vi "WPI_AccumulatorToVoltageSeconds.vi"(8 "error in (no error)":errorcluster, 10 "Value":i64, 11 "AIDeviceRef":T1={"DevStatus"={"status"=FALSE, "code"=0, "source"=""}, "Analog Channel"=enum."AI 1"}) -> (0 "error out":errorcluster, 2 "Volt Seconds":dbl, 3 "AIDeviceRef":T1={"DevStatus"={"status"=FALSE, "code"=0, "source"=""}, "Analog Channel"=enum."AI 1"})   [LabVIEW 2017]
uses:
  <vilib>/Rock Robotics/WPI/AnalogChannel/WPI_AnalogChannelDevRef.ctl
  <vilib>/Rock Robotics/SystemInterfaces/AI/FPGA_AIChannel.ctl
  <vilib>/Rock Robotics/SystemInterfaces/System/FPGA_SystemGet.vi
  <vilib>/Rock Robotics/SystemInterfaces/AI/FPGA_AIAverageBits.vi
  <vilib>/Rock Robotics/SystemInterfaces/AI/FPGA_AIERRInvalidAnalogChannel.vi
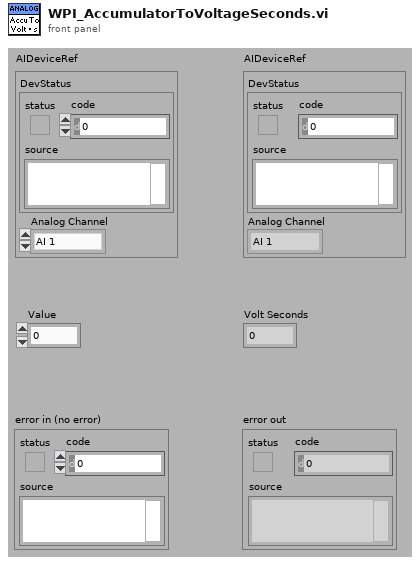
[diagram p1: front panel]
types:
  T1 = typedef "WPI_AnalogChannelDevRef.ctl" = cluster{"DevStatus":errorcluster, "Analog Channel":T2}
  T2 = typedef "FPGA_AIChannel.ctl" = enum8{"AI 0", "AI 1", "AI 2", "AI 3", "AI MXP 0", "AI MXP 1", "AI MXP 2", "AI MXP 3", "Invalid"}
  T3 = typedef "FPGA_AIDevRef.ctl" = cluster{"DevStatus":errorcluster}
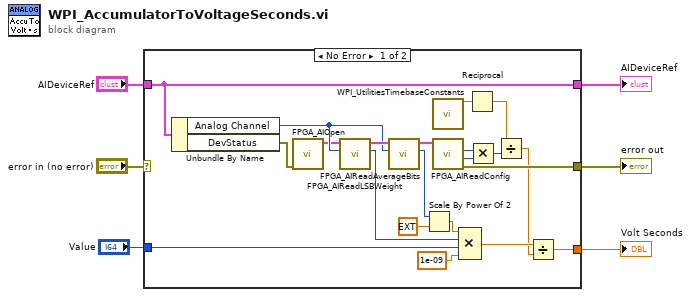
[diagram p0: block diagram]
diagram:
  n1 = case shown="No Error" "error in (no error)" {
    selector: "error in (no error)" -> [_ w29]
    tunnel: "Value" -> [w9 _]
    tunnel: "AIDeviceRef" -> [w7 w28]
    tunnel: [w7 w28] -> w3
    tunnel: [w13 w29] -> w2
    tunnel: [w10 _] -> w1
    frame No Error {
      n2 = Unbundle By Name(w7) -> ("Analog Channel"=w22:T2, "DevStatus"=w26:errorcluster)
      n3 = call <vilib>:"FPGA_AIOpen.vi"("error in (no error)"=w26) -> ("AI Reference out"=w19:T3)  [unwired: 2 in, 8 out]
      n4 = call <vilib>:"FPGA_AIReadLSBWeight.vi"("Channel"=w22, "AI Reference"=w19) -> ("LSBWeight"=w24:u32, "AI Reference"=w23:T3)  [unwired: 1 in, 7 out]
      n5 = call <vilib>:"FPGA_AIReadAverageBits.vi"("Channel"=w22, "AI Reference in"=w23) -> ("AverageBits"=w21:u8, "AI Reference out"=w14:T3)  [unwired: 1 in, 7 out]
      n6 = Scale By Power Of 2(n=w21, x=ext 1.0) -> (x*2^n=w20:ext)
      n7 = call <vilib>:"WPI_UtilitiesTimebaseConstants.vi"() -> ("40 MHz FPGA clock"=w17:dbl)  [unwired: 13 in, 2 out]
      n8 = call <vilib>:"FPGA_AIReadConfig.vi"("AI Reference"=w14) -> ("error out"=w13:errorcluster, "Convert Rate"=w15:u32, "Scan Size"=w16:u8)  [unwired: 1 in, 7 out]
      n9 = Compound Arithmetic op=MULTIPLY(w20, w24, w9, 1e-09 ("y")) -> (w12:ext)
      n10 = Reciprocal(x=w17) -> (1/x=w8:dbl)
      n11 = Multiply(x=w16, y=w15) -> (x*y=w18:u32)
      n12 = Divide(x=w8, y=w18) -> (x/y=w11:dbl)
      n13 = Divide(x=w12, y=w11) -> (x/y=w10:ext)
    }
    frame Error {
    }
  }
  "Volt Seconds" <- w1
  "error out" <- w2
  "AIDeviceRef" <- w3
